vi "Get List of TestCases.vi"(8 "error in (no error)":errorcluster, 10 "Filter":T1, 11 "Pips in":refnum<class "Pips.lvclass">) -> (0 "error out":errorcluster, 2 "TestCases":string[](array[string]), 3 "Pips out":refnum<class "Pips.lvclass">)   [LabVIEW 2021, in "Bananas.lvlib" / "Pips.lvclass"]
uses:
  Pips.lvclass
  pip_filter -- enum.ctl
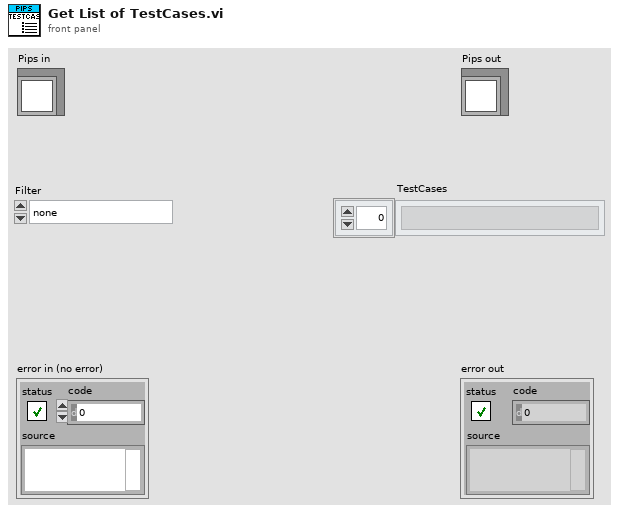
[diagram p1: front panel]
types:
  T1 = typedef "Bananas.lvlib/Pips.lvclass/pip_filter -- enum.ctl" = enum16{"none", "passed", "skipped", "covered", "uncovered"}
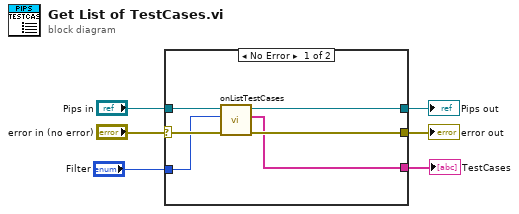
[diagram p0: block diagram]
diagram:
  n1 = case shown="No Error" "error in (no error)" {
    selector: "error in (no error)" -> [w10 w14]
    tunnel: [w9 w14] -> w5
    tunnel: [w11 w13] -> w3
    tunnel: "Pips in" -> [w12 w13]
    tunnel: "Filter" -> [w7 _]
    tunnel: [w8 _] -> w1
    frame No Error {
      n2 = call-dynamic "onListTestCases.vi"("error in (no error)"=w10, "Filter"=w7, "Pips in"=w12) -> ("error out"=w9:errorcluster, "TestCases"=w8:string[], "Pips out"=w11:refnum<class "Pips.lvclass">)  [unwired: 6 in]
    }
    frame Error {
    }
  }
  "error out" <- w5
  "Pips out" <- w3
  "TestCases" <- w1
